vi "SMO.Activity.SetActivityManager.vi"(8 "error in (no error)":errorcluster, 11 "SMO.Activity in":refnum<class "SMO.Activity.lvclass">) -> (0 "error out":errorcluster, 3 "SMO.Activity out":refnum<class "SMO.Activity.lvclass">)   [LabVIEW 2015, in "SMO.Activity.lvclass"]
uses:
  SMO.Activity.lvclass
  <vilib>/JKI/JKI SMO/SMO/SMO.lvclass
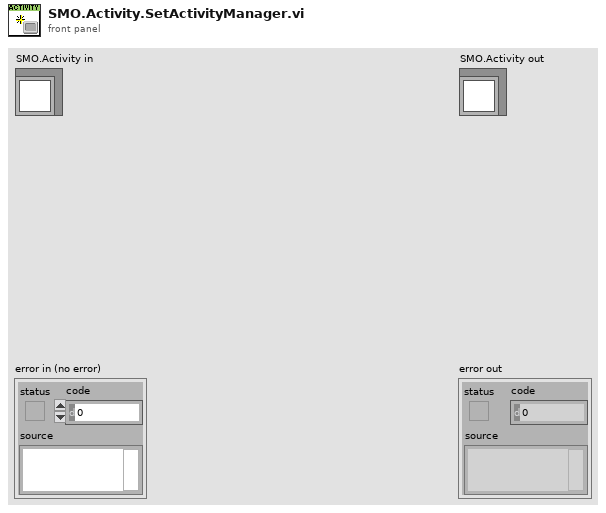
[diagram p1: front panel]
types:
  T1 = typedef "SMO.Activity.lvclass/PrivateData--Ref.ctl" = refnum<data-value>
  T2 = typedef "SMO.Activity.lvclass/PrivateData--Cluster.ctl" = cluster{"Public Events":T3, "Subpanel Ref":refnum<vi>, "UI State":T4}
  T3 = typedef "SMO.Activity.lvclass/PublicEvents--Cluster.ctl" = cluster{"UI State":refnum<user-event>}
  T4 = typedef "SMO.Activity.lvclass/SMO.UI_Embed State--enum.ctl" = enum16{"unknown", "Opened", "Embedded", "Closed"}
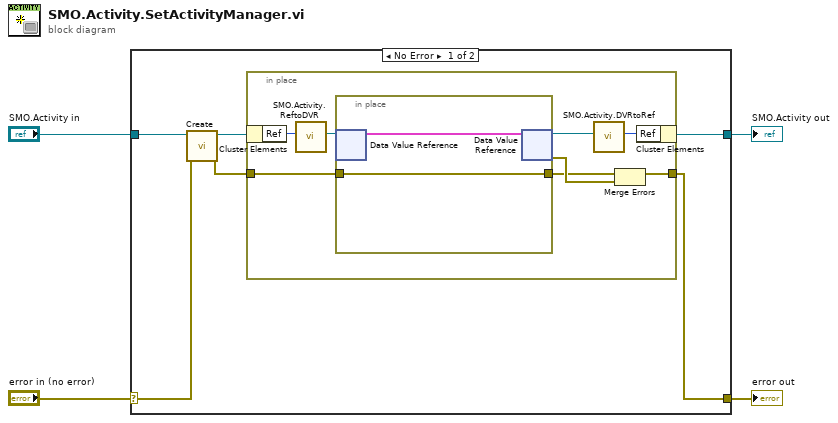
[diagram p0: block diagram]
diagram:
  n1 = case shown="No Error" "error in (no error)" {
    selector: "error in (no error)" -> [w9 w22]
    tunnel: [w5 w22] -> w3
    tunnel: [w7 w21] -> w1
    tunnel: "SMO.Activity in" -> [w10 w21]
    frame No Error {
      n2 = call <vilib>:"Create.vi"("error in (no error)"=w9, "SMO"=w10) -> ("error out"=w6:errorcluster, "SMO out"=w8:refnum<class "SMO.Activity.lvclass">)  [unwired: 7 in, 1 out]
      n3 = in-place {
        in-place-border: w6 -> [w18]
        in-place-border: [w15] -> w5
        n4 = in-place-cluster #1(w8) -> ("Ref"=w12:u32)
        n5 = call "SMO.Activity.ReftoDVR.vi"("Ref"=w12) -> ("Ref"=w11:T1)  [unwired: 10 in]
        n6 = in-place {
          in-place-border: w18 -> [w20]
          in-place-border: [w20] -> w16
          n7 = in-place-dvr #2(w11) -> (w19:T2)  [unwired: 1 out]
          n8 = in-place-dvr #2(w19) -> (w14:T1, w17:errorcluster)
        }
        n9 = call "SMO.Activity.DVRtoRef.vi"("Ref"=w14) -> ("Ref"=w13:u32)  [unwired: 10 in]
        n10 = Merge Errors(w16, w17) -> (w15:errorcluster)
        n11 = in-place-cluster #1("Ref"=w13) -> (w7:refnum<class "SMO.Activity.lvclass">)
      }
    }
    frame Error {
    }
  }
  "error out" <- w3
  "SMO.Activity out" <- w1
